vi "Actor Framework Top Level.vi"() -> ()   [LabVIEW 2020]
uses:
  DMM Actor/DMM Driver.lvclass
  C:/Program Files (x86)/National Instruments/LabVIEW 2020/vi.lib/ActorFramework/Actor/Actor.lvclass
  <vilib>/ActorFramework/Message Queue/Message Queue.lvclass/Message Queue.ctl
  <vilib>/ActorFramework/Message Queue/Message Queue.lvclass
  <vilib>/ActorFramework/Actor/Actor.lvclass
panel:
  out "error out":errorcluster
  in  "error in (no error)":errorcluster
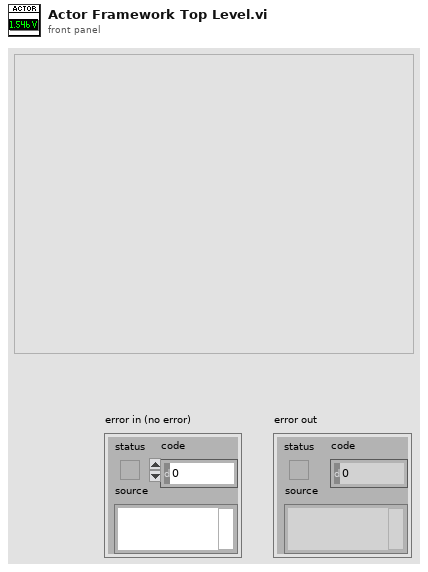
[diagram p1: front panel]
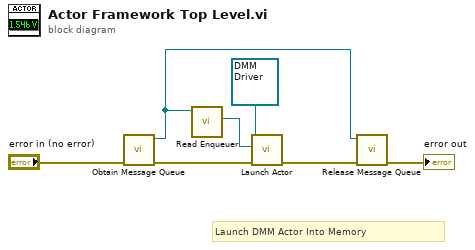
[diagram p0: block diagram]
diagram:
  # "Launch DMM Actor Into Memory"
  n1 = call <vilib>:"Obtain Message Queue.vi"("error in (no error)"="error in (no error)") -> ("error out"=w6:errorcluster, "Message Queue"=w4:refnum<class "Message Queue.lvclass">)  [unwired: 9 in]
  n2 = call <vilib>:"Read Enqueuer.vi"("Message Queue"=w4) -> ("Message Enqueuer"=w5:refnum<class "Message Enqueuer.lvclass">)  [unwired: 10 in]
  n3 = call <vilib>:"Launch Actor.vi"("error in (no error)"=w6, "Actor-to-Caller Enqueuer"=w5, "Actor"=refnum<class "DMM Driver.lvclass"> refnum ("DMM Driver.lvclass")) -> ("error out"=w7:errorcluster)  [unwired: 7 in, 1 out]
  n4 = call <vilib>:"Release Message Queue.vi"("error in (no error)"=w7, "Message Queue"=w4) -> ("error out"=→"error out":errorcluster)  [unwired: 8 in, 1 out]
